vi "Hide Label & Caption when Running.vi"(10 "Container State":T1, 11 "Display State out in":T2={"Window Handle"=refnum, "Maximum"=0, "State Change Action"=enum."Method - Initialize", "Running"=FALSE, "Visable Items"={"Label"=TRUE, "Caption"=FALSE}, "Value"=100, "Show Progress Bar"=FALSE} caption="State") -> (3 "Display State out out":T2={"Window Handle"=refnum, "Maximum"=0, "State Change Action"=enum."Method - Initialize", "Running"=FALSE, "Visable Items"={"Label"=TRUE, "Caption"=FALSE}, "Value"=100, "Show Progress Bar"=FALSE} caption="State")   [LabVIEW 2011, in "Taskbar Progress Bar.xctl"]
uses:
  Taskbar Progress Bar.xctl
  Abilities/TPB State.ctl
  TypeDefs/Dispaly State Change Methods.ctl
  <vilib>/_xctls/Container State.ctl
  <vilib>/_xctls/XControlSupport.lvlib
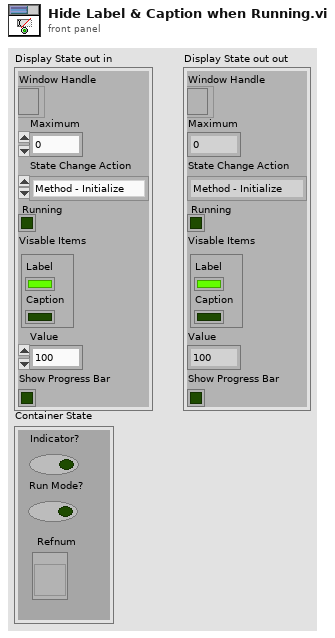
[diagram p1: front panel]
types:
  T1 = typedef "XControlSupport.lvlib/Container State.ctl" = cluster{"Indicator?":bool, "Run Mode?":bool, " Refnum":refnum<vi>}
  T2 = typedef "Taskbar Progress Bar.xctl/TPB State.ctl" = cluster{"Window Handle":refnum<k24>, "Maximum":u64, "State Change Action":T3, "Running":bool, "Visable Items":cluster{"Label":bool, "Caption":bool}, "Value":u64, "Show Progress Bar":bool}
  T3 = typedef "Taskbar Progress Bar.xctl/Dispaly State Change Methods.ctl" = enum16{"No Action", "Created", "Method - Initialize", "Method - Increment", "Method - Set Value", "Method - Pause", "Method - Error", "Method - Finish", "Property - Show Progress Bar"}
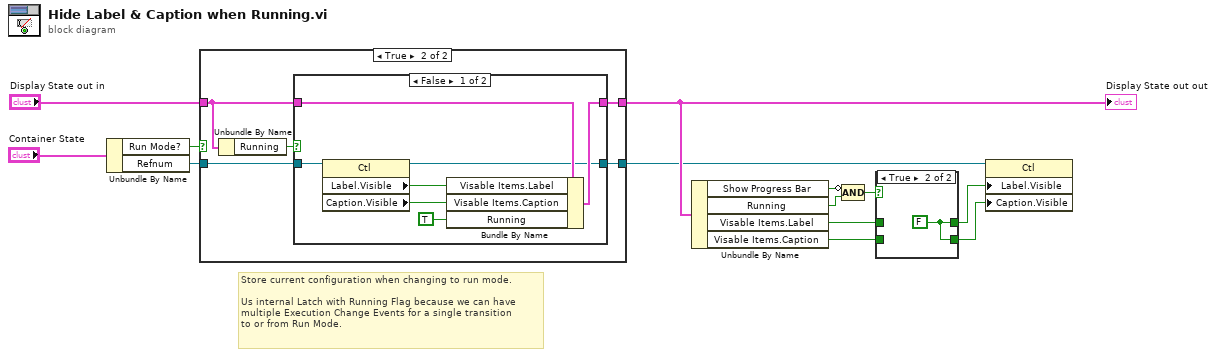
[diagram p0: block diagram]
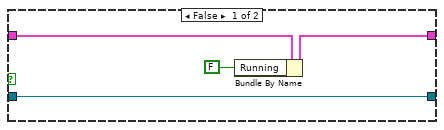
[diagram p3: hidden frame]
diagram:
  # "Store current configuration when changing to run mode.\n\nUs internal Latch with Running Flag because we can have\nmultiple Execution Change Events for a single transition\nto or from Run Mode."
  n1 = Unbundle By Name("Container State") -> ("Run Mode?"=w10:bool, "Refnum"=w11:refnum<vi>)
  n2 = case shown="True" w10 {
    tunnel: "Display State out in" -> [w16 w18]
    tunnel: w11 -> [w17 w22]
    tunnel: [w15 w21] -> w9
    tunnel: [w17 w20] -> w6
    frame False {
      n3 = Bundle By Name(cluster=w16, "Running"=FALSE) -> (w15:T2)
    }
    frame True {
      n4 = Unbundle By Name(w18) -> ("Running"=w19:bool)
      n5 = case shown="False" w19 {
        tunnel: w22 -> [w29 w31]
        tunnel: w18 -> [w26 w30]
        tunnel: [w25 w30] -> w21
        tunnel: [w24 w31] -> w20
        frame False {
          n6 = property class="Ctl"(reference=w29) -> (reference out=w24:refnum<vi>, "Label.Visible"=w28:bool, "Caption.Visible"=w27:bool)  [unwired: 1 in, 1 out]
          n7 = Bundle By Name(cluster=w26, "Visable Items.Label"=w28, "Visable Items.Caption"=w27, "Running"=TRUE) -> (w25:T2)
        }
        frame True {
        }
      }
    }
  }
  "Display State out out" <- w9
  n8 = Unbundle By Name(w9) -> ("Show Progress Bar"=w3:bool, "Running"=w2:bool, "Visable Items.Label"=w8:bool, "Visable Items.Caption"=w7:bool)
  n9 = Compound Arithmetic op=AND(invert w3, w2) -> (w1:bool)
  n10 = case shown="True" w1 {
    tunnel: w8 -> [w33 _]
    tunnel: [w33 w34] -> w5
    tunnel: [w32 w34] -> w4
    tunnel: w7 -> [w32 _]
    frame False {
    }
    frame True {
      w34 = FALSE ("Label")
    }
  }
  n11 = property class="Ctl"(reference=w6, "Label.Visible"=w5, "Caption.Visible"=w4) -> ()  [unwired: 1 in, 2 out]
